vi "App Reference FGV.vi"(7 "Mode":T1, 8 "error in (no error)":errorcluster, 11 "App Ref":refnum<vi>) -> (0 "error out":errorcluster, 3 "App Ref out":refnum<vi>)   [LabVIEW 2020, in "MacroAssert.lvlib"]
doc: "FGV for setting, starting, and reading a timer."
uses:
  MacroAssert.lvlib
  CTLs/FGV Actions.ctl
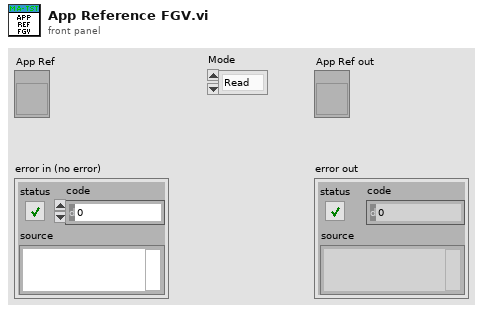
[diagram p1: front panel]
types:
  T1 = typedef "MacroAssert.lvlib/FGV Actions.ctl" = enum16{"Read", "Write"}
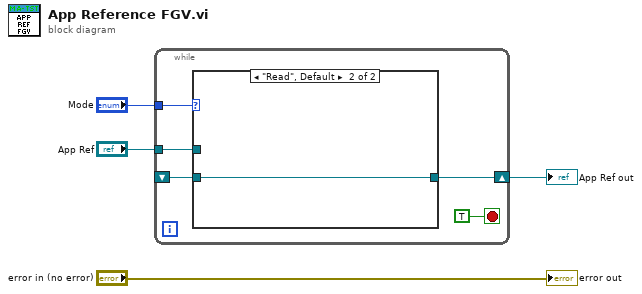
[diagram p0: block diagram]
diagram:
  n1 = while {
    tunnel: "Mode" -> [w9]
    shift-right: [w6] -> w1
    shift-left: _ -> [w7]
    tunnel: "App Ref" -> [w5]
    stop <- TRUE stop-if-true
    n2 = case shown="\"Read\", Default" w9 {
      tunnel: w7 -> [_ w11]
      tunnel: [w10 w11] -> w6
      tunnel: w5 -> [w10 _]
      frame "Write" {
      }
      frame "Read", Default {
      }
    }
  }
  "App Ref out" <- w1
  "error out" <- "error in (no error)"
